vi "3.1-Act Arbitrator.vi"() -> ()   [LabVIEW 2010]
uses:
  2-Low Neurons/2.1 PID Gains Typedef.ctl
  2-Low Neurons/2.1-Act Command Typedef.ctl
  <vilib>/rvi/interface/nirviReadWriteControl/nirviReadWriteControl.xnode
  2-Low Neurons/2-FPGA VI Typedef.ctl
  FPGA Bitfiles/DaveBrain_FPGATarget_1-Hindbrain_F0E489D8.lvbitx
  1-Hindbrain.vi
  <vilib>/rvi/interface/common/niFpgaNodeNameForErrorReporting.ctl
  <vilib>/rvi/errors/niLvFpgaWhatHappensToTopLevelVI.ctl
  3.0-Global.vi
  <vilib>/Utility/error.llb/Error Cluster From Error Code.vi
  <vilib>/rvi/errors/niLvFpgaAdjustHostInterfaceError.vi
  NiFpgaLv.dll
panel:
  in  "ticks per degree":dbl=300.0
  in  "magic zero point number":i32
  in  "2.1.3 Drive PID Gains":T1={"P Gain"=0.25, "I Gain"=0.25, "D Gain"=0.25, "P Gain - Exp"=2, "I Gain - Exp"=2, "D Gain - Exp"=2, "I Saturate"=0.25} {"I Saturate" format="%#_14g"; "P Gain" format="%.8f"; "I Gain" format="%.8f"; "D Gain" format="%.8f"}
  in  "2.1.3 Lidar PID Gains":T1={"P Gain"=0.25, "I Gain"=0.25, "D Gain"=0.25, "P Gain - Exp"=2, "I Gain - Exp"=2, "D Gain - Exp"=2, "I Saturate"=0.25} {"I Saturate" format="%#_14g"; "P Gain" format="%.8f"; "I Gain" format="%.8f"; "D Gain" format="%.8f"}
  in  "2.1.3 Steering PID Gains":T1={"P Gain"=0.25, "I Gain"=0.25, "D Gain"=0.25, "P Gain - Exp"=2, "I Gain - Exp"=2, "D Gain - Exp"=2, "I Saturate"=0.25} {"I Saturate" format="%#_14g"; "P Gain" format="%.8f"; "I Gain" format="%.8f"; "D Gain" format="%.8f"}
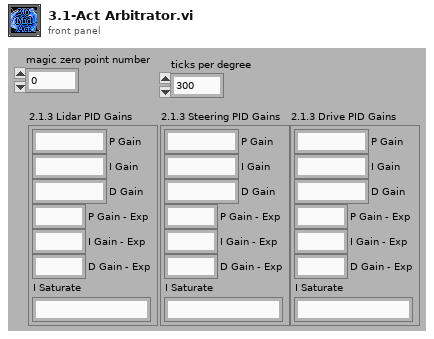
[diagram p1: front panel]
types:
  T1 = typedef "2.1 PID Gains Typedef.ctl" = cluster{"P Gain":fxp<+/-,18,1>, "I Gain":fxp<+/-,18,1>, "D Gain":fxp<+/-,18,1>, "P Gain - Exp":i8, "I Gain - Exp":i8, "D Gain - Exp":i8, "I Saturate":fxp<+/-,64,46>}
  T2 = typedef "2.1-Act Command Typedef.ctl" = cluster{"Inhibit All Motors":bool, "2.1 Direct Override":bool, "Drive Speed Integer Setpoint":i32, "Steering Integer Setpoint":i32, "Lidar Position Integer Setpoint":i32, "Drive Direct":fxp<+/-,20,5>, "Steer Direct":fxp<+/-,20,5>, "Lidar Direct ":fxp<+/-,20,5>, "2.1.3 Drive PID Gains":T1, "2.1.3 Steering PID Gains":T1, "2.1.3 Lidar PID Gains":T1, "2.5.5 A":fxp<+/-,18,1>, "2.5.6 B":fxp<+/-,18,1>, "Drive Limit":fxp<+/-,20,5>}
  T3 = typedef "niFpgaNodeNameForErrorReporting.ctl" = enum16{"Open FPGA VI Reference", "Read/Write Control", "Invoke Method: Abort", "Invoke Method: Acknowledge IRQ", "Invoke Method: Download", "Invoke Method: FIFO.Configure", "Invoke Method: FIFO.Read", "Invoke Method: FIFO.Start", "Invoke Method: FIFO.Stop", "Invoke Method: FIFO.Write", "Invoke Method: Reset", "Invoke Method: Run", "Invoke Method: Wait on IRQ", "Close FPGA VI Reference"}
  T4 = typedef "niLvFpgaWhatHappensToTopLevelVI.ctl" = enum16{"top level VI scripted behind XNode", "top level VI inlined behind XNode"}
  T5 = typedef "4.1.2-Act Neuron TD.ctl" = cluster{"Speed By Path":dbl[]}
  T6 = typedef "2-FPGA VI Typedef.ctl" = refnum<k20>
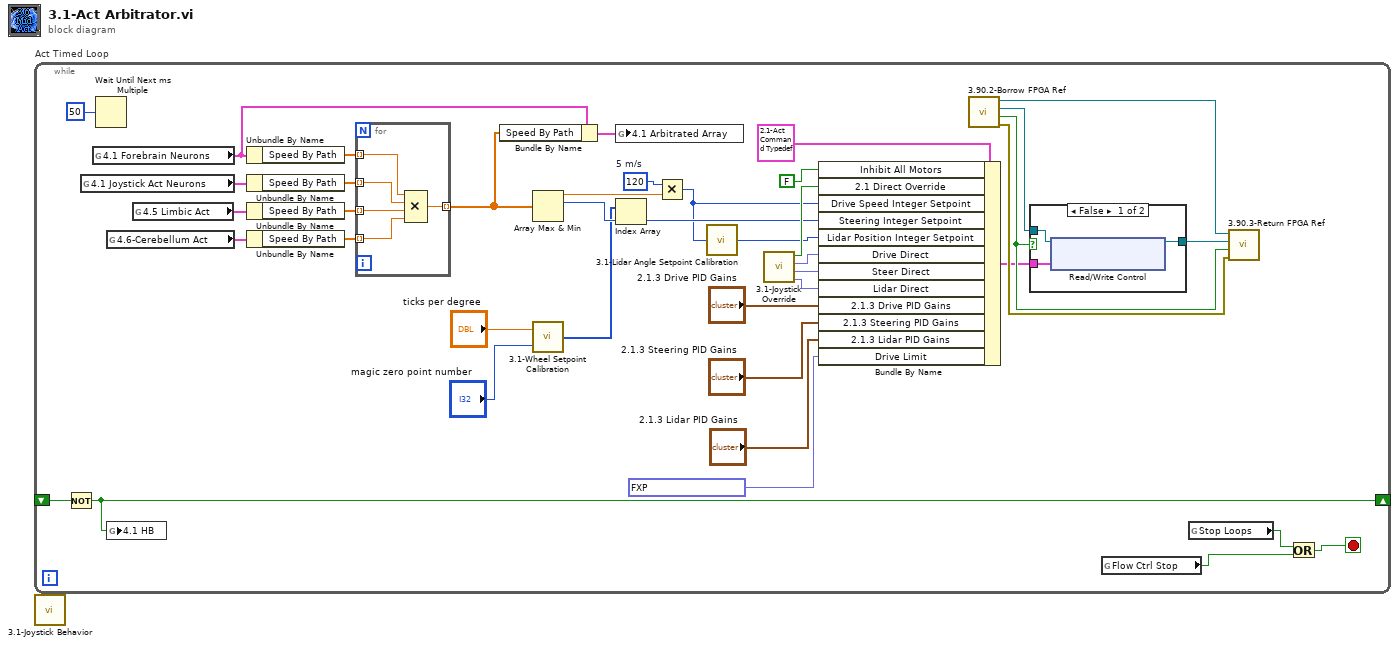
[diagram p0: block diagram]
diagram:
  n1 = while "Act Timed Loop" {
    shift-right: [w33] -> _
    shift-left: _ -> [w41]
    stop <- w1 stop-if-true
    w12 = 120  # 5 m/s
    n2 = Not(x=w41) -> (.not. x?=w33:bool)
    n3 = global read "3.0-Global.vi" "4.1 Joystick Act Neurons"() -> (w26:T5)
    n4 = global read "3.0-Global.vi" "4.1 Forebrain Neurons"() -> (w15:T5)
    n5 = Wait Until Next ms Multiple(millisecond multiple=u32 50) -> ()  [unwired: 1 out]
    n6 = global read "3.0-Global.vi" "4.6-Cerebellum Act"() -> (w28:T5)
    n7 = global write "3.0-Global.vi" "4.1 HB"(w33) -> ()
    n8 = global read "3.0-Global.vi" "4.5 Limbic Act"() -> (w27:T5)
    n9 = Unbundle By Name(w15) -> ("Speed By Path"=w29:dbl[])
    n10 = Unbundle By Name(w26) -> ("Speed By Path"=w25:dbl[])
    n11 = Unbundle By Name(w27) -> ("Speed By Path"=w24:dbl[])
    n12 = Unbundle By Name(w28) -> ("Speed By Path"=w23:dbl[])
    n13 = for {
      tunnel: w29 -> [w46] mode=indexing
      tunnel: w25 -> [w45] mode=indexing
      tunnel: w24 -> [w44] mode=indexing
      tunnel: w23 -> [w43] mode=indexing
      tunnel: [w42] -> w13 mode=indexing
      n14 = Compound Arithmetic op=MULTIPLY(w46, w45, w44, w43) -> (w42:dbl)
    }
    n15 = Bundle By Name(cluster=w15, "Speed By Path"=w13) -> (w14:T5)
    n16 = Array Max & Min(array=w13) -> (max value=w11:dbl, max index (indices)=w10:i32)  [unwired: 2 out]
    n17 = call "3.1-Wheel Setpoint Calibration.vi"("magic zero point number"="magic zero point number", "ticks per degree"="ticks per degree") -> ("Array"=w6:i32[])
    n18 = global write "3.0-Global.vi" "4.1 Arbitrated Array"(w14) -> ()
    n19 = Index Array(array=w6, index=w10) -> (element=w9:i32)
    n20 = Multiply(x=w12, y=w11) -> (x*y=w4:i32)
    n21 = call "3.1-Lidar Angle Setpoint Calibration.vi"("Numeric"=w4) -> ("Numeric 2"=w5:i32)
    n22 = call "3.1-Joystick Override.vi"() -> ("Numeric"=w16:fxp<+/-,19,4>, "Numeric 2"=w17:fxp<+/-,19,4>, "Numeric 3"=w18:fxp<+/-,19,4>, "Trig"=w30:bool)
    n23 = Bundle By Name(cluster=T2 {"Inhibit All Motors"=FALSE, "2.1 Direct Override"=FALSE, "Drive Speed Integer Setpoint"=0, "Steering Integer Setpoint"=0, "Lidar Position Integer Setpoint"=0, "Drive Direct"=0.0, "Steer Direct"=0.0, "Lidar Direct "=0.0, "2.1.3 Drive PID Gains"={"P Gain"=0.0, "I Gain"=0.0, "D Gain"=0.0, "P Gain - Exp"=0, "I Gain - Exp"=0, "D Gain - Exp"=0, "I Saturate"=0.0}, "2.1.3 Steering PID Gains"={"P Gain"=0.0, "I Gain"=0.0, "D Gain"=0.0, "P Gain - Exp"=0, "I Gain - Exp"=0, "D Gain - Exp"=0, "I Saturate"=0.0}, "2.1.3 Lidar PID Gains"={"P Gain"=0.0, "I Gain"=0.0, "D Gain"=0.0, "P Gain - Exp"=0, "I Gain - Exp"=0, "D Gain - Exp"=0, "I Saturate"=0.0}, "2.5.5 A"=0.0, "2.5.6 B"=0.0, "Drive Limit"=0.0} ("2.1 Act Command"), "Inhibit All Motors"=FALSE, "2.1 Direct Override"=w30, "Drive Speed Integer Setpoint"=w4, "Steering Integer Setpoint"=w9, "Lidar Position Integer Setpoint"=w5, "Drive Direct"=w18, "Steer Direct"=w17, "Lidar Direct"=w16, "2.1.3 Drive PID Gains"="2.1.3 Drive PID Gains", "2.1.3 Steering PID Gains"="2.1.3 Steering PID Gains", "2.1.3 Lidar PID Gains"="2.1.3 Lidar PID Gains", "Drive Limit"=fxp<+/-,20,5> 5.0) -> (w34:T2)
    n24 = call "3.90.2-Borrow FPGA Ref.vi"() -> ("error out"=w39:errorcluster, "Failed to Obtain Ref"=w37:bool, "element"=w38:T6, "FPGA Ref"=w40:refnum<queue>)  [unwired: 4 in]
    n25 = case shown="False" w37 {
      tunnel: w38 -> [w49 w93]
      tunnel: [w48 w93] -> w36
      tunnel: w34 -> [w47 _]
      frame False {
        n26 = xnode "Read/Write Control"("FPGA VI Reference In"=w49, "2.1 Act Command"=w47) -> ("FPGA VI Reference Out"=w48:T6)  [unwired: 1 in, 1 out]
      }
      frame True {
      }
    }
    n27 = global read "3.0-Global.vi" "Flow Ctrl Stop"() -> (w2:bool)
    n28 = global read "3.0-Global.vi" "Stop Loops"() -> (w3:bool)
    n29 = call "3.90.3-Return FPGA Ref.vi"("error in"=w39, "Failed to Obtain Ref"=w37, "element"=w36, "FPGA Ref"=w40) -> ()  [unwired: 1 out]
    n30 = Or(x=w3, y=w2) -> (x .or. y?=w1:bool)
  }
  n31 = call "3.1-Joystick Behavior.vi"() -> ()  [unwired: 12 in]
